vi "6 Type Casting.vi"() -> ()   [LabVIEW 2015]
panel:
  in  "Knob":i8(knob) min=0 max=100 step=5 scale=0.0..100.0
  in  "stop":bool
  out "SUM":u16
  in  "X (integer)":u8 max=100 step=5
  in  "X (double)":u8 max=100 step=5
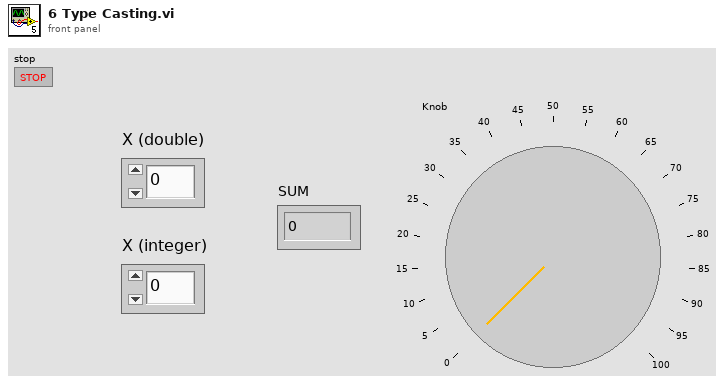
[diagram p1: front panel]
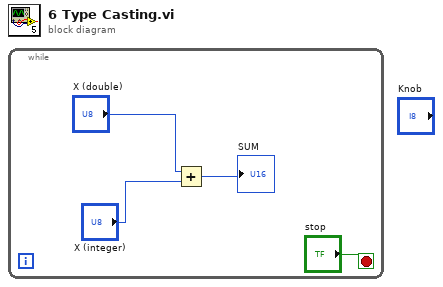
[diagram p0: block diagram]
diagram:
  n1 = while {
    stop <- "stop" stop-if-true
    n2 = Add(x="X (double)", y="X (integer)") -> (x+y=→"SUM":u8)
  }
